vi "mirrorOutput.vi"() -> ()   [LabVIEW 2015]
uses:
  <vilib>/rvi/Emulation/niFpgaGetClockAttributes.vi
  <vilib>/rvi/Emulation/niFpgaSctlEmulationGetInTimedLoop.vi
  <vilib>/rvi/Emulation/niFpgaEmulationReportErrorSimple.vi
  <vilib>/rvi/interface/RandomDataEmulation/nirviRandomDataMultiElementFPGAFIFO.vi
  <instcachedir>/0/nirviRandomDataMultiElementFPGAFIFO_0B1D92D8D7EE43F2AC2E0B59792129FA.lvgen/nirviRandomDataMultiElementFPGAFIFO_0B1D92D8D7EE43F2AC2E0B59792129FA_003.vi
  <vilib>/rvi/interface/RandomDataEmulation/niFpgaRandomDataHandleErrors.vi
  <vilib>/rvi/eio/common/nirviEmuTemplateMethod_errors.vi
  <vilib>/rvi/Emulation/niFpgaCriticalErrorInLSC.vi
  <vilib>/rvi/DataTransferAndStorage/Container/XNode/niFpgaContainer.xnode
  <vilib>/rvi/interface/RandomDataEmulation/nirviRandomDataFpgaMultiElementTemplate.vi
  <vilib>/eio/EIONode/EIONode.xnode
panel:
  in  "stop":bool
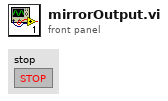
[diagram p1: front panel]
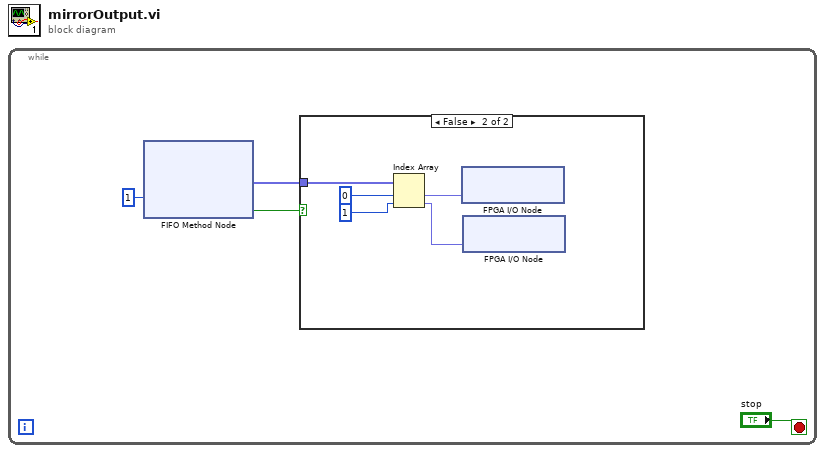
[diagram p0: block diagram]
diagram:
  n1 = while {
    stop <- "stop" stop-if-true
    n2 = xnode ("FIFO Method Node")("Timeout"=1) -> ("Element"=w4:fxp<+/-,20,5>[], "Timed Out?"=w1:bool)  [unwired: 1 in, 1 out]
    n3 = case shown="False" w1 {
      tunnel: w4 -> [_ w9]
      frame True {
      }
      frame False {
        n4 = Index Array(array=w9, index #1=0 ("index"), index #2=1 ("length")) -> (element #1=w6:fxp<+/-,20,5>, element #2=w5:fxp<+/-,20,5>)
        n5 = xnode "FPGA I/O Node"("Mod5/AO2"=w6) -> ()  [unwired: 1 in, 1 out]
        n6 = xnode "FPGA I/O Node"("Mod5/AO3"=w5) -> ()  [unwired: 1 in, 1 out]
      }
    }
  }
